vi "Lire Stocks.vi"(11 "Portfolio en entrée":refnum<class "Portfolio.lvclass">) -> (2 "Stocks":refnum<class "Stock.lvclass">[](array[class]), 3 "Portfolio en sortie":refnum<class "Portfolio.lvclass">)   [LabVIEW 2012, in "Portfolio.lvclass"]
uses:
  Portfolio.lvclass
  Stock/Stock.lvclass
  Portfolio.lvclass/Portfolio.ctl
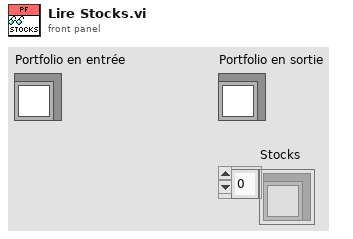
[diagram p1: front panel]
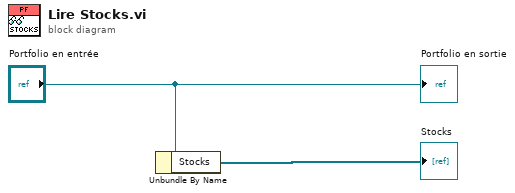
[diagram p0: block diagram]
diagram:
  n1 = Unbundle By Name("Portfolio en entrée") -> ("Stocks"=→"Stocks":refnum<class "Stock.lvclass">[])
  "Portfolio en sortie" <- "Portfolio en entrée"
